vi "Data.Engine.Resize.vi"(8 "error in":errorcluster, 11 "Data Access API in":refnum<class "Data Access Engine.lvclass">) -> (0 "error out":errorcluster, 3 "Data Access API out":refnum<class "Data Access Engine.lvclass">)   [LabVIEW 2023, in "Data Access Engine.lvlib" / "Data Access Engine.lvclass"]
uses:
  Data Access Engine.lvclass
  Data Access Engine.lvclass/Data Access Engine.ctl
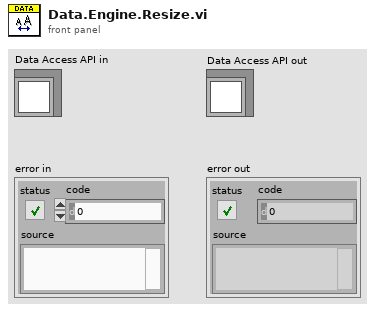
[diagram p1: front panel]
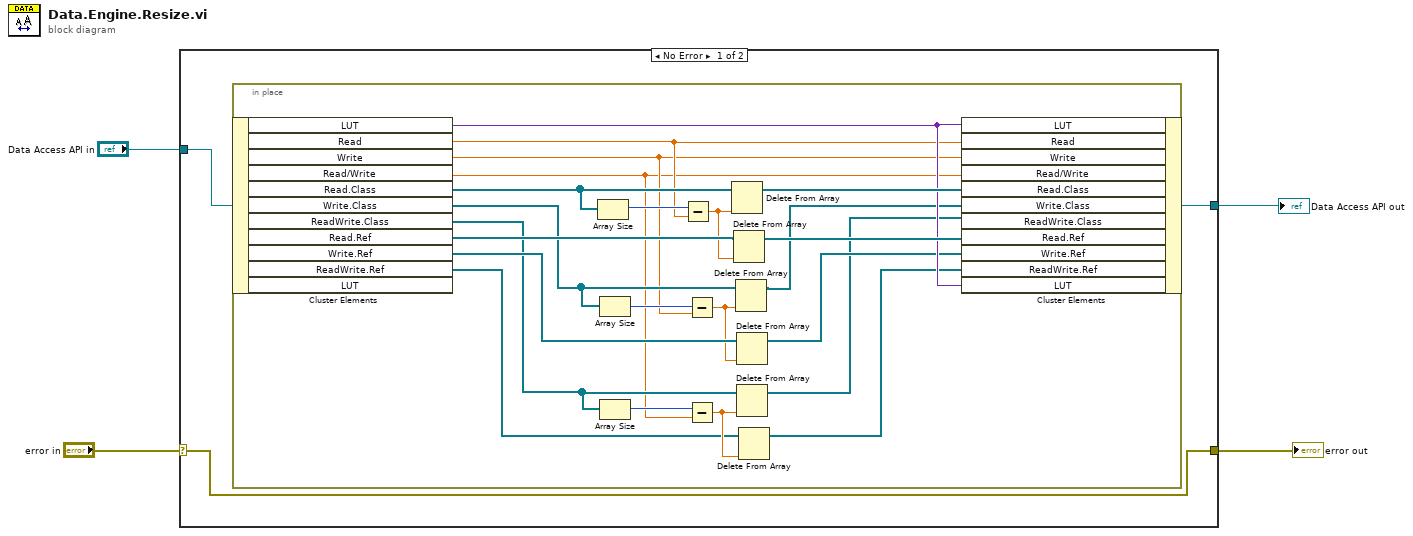
[diagram p0: block diagram]
diagram:
  n1 = case shown="No Error" "error in" {
    selector: "error in" -> [w7 w31]
    tunnel: "Data Access API in" -> [w6 w30]
    tunnel: [w7 w31] -> w3
    tunnel: [w5 w30] -> w1
    frame No Error {
      n2 = in-place {
        n3 = in-place-cluster #1(w6) -> ("LUT"=w24:variant, "Read"=w10:dbl, "Write"=w9:dbl, "Read/Write"=w8:dbl, "Read.Class"=w29:refnum<class "Read.lvclass">[], "Write.Class"=w23:refnum<class "Write.lvclass">[], "ReadWrite.Class"=w14:refnum<class "ReadWrite.lvclass">[], "Read.Ref"=w26:refnum<data-value>[], "Write.Ref"=w20:refnum<data-value>[], "ReadWrite.Ref"=w12:refnum<data-value>[])  [unwired: 1 out]
        n4 = Array Size(array=w29) -> (size(s)=w28:i32)
        n5 = Array Size(array=w23) -> (size(s)=w21:i32)
        n6 = Array Size(array=w14) -> (size(s)=w15:i32)
        n7 = Subtract(x=w28, y=w10) -> (x-y=w22:dbl)
        n8 = Subtract(x=w21, y=w9) -> (x-y=w18:dbl)
        n9 = Subtract(x=w15, y=w8) -> (x-y=w13:dbl)
        n10 = Delete From Array(array=w29, index=w22) -> (array with subset deleted=w27:refnum<class "Read.lvclass">[])  [unwired: 1 in, 1 out]
        n11 = Delete From Array(array=w26, index=w22) -> (array with subset deleted=w25:refnum<data-value>[])  [unwired: 1 in, 1 out]
        n12 = Delete From Array(array=w23, index=w18) -> (array with subset deleted=w16:refnum<class "Write.lvclass">[])  [unwired: 1 in, 1 out]
        n13 = Delete From Array(array=w20, index=w18) -> (array with subset deleted=w19:refnum<data-value>[])  [unwired: 1 in, 1 out]
        n14 = Delete From Array(array=w14, index=w13) -> (array with subset deleted=w17:refnum<class "ReadWrite.lvclass">[])  [unwired: 1 in, 1 out]
        n15 = Delete From Array(array=w12, index=w13) -> (array with subset deleted=w11:refnum<data-value>[])  [unwired: 1 in, 1 out]
        n16 = in-place-cluster #1("LUT"=w24, "Read"=w10, "Write"=w9, "Read/Write"=w8, "Read.Class"=w27, "Write.Class"=w16, "ReadWrite.Class"=w17, "Read.Ref"=w25, "Write.Ref"=w19, "ReadWrite.Ref"=w11, "LUT"=w24) -> (w5:refnum<class "Data Access Engine.lvclass">)
      }
    }
    frame Error {
    }
  }
  "error out" <- w3
  "Data Access API out" <- w1
